vi "Main.vi"() -> ()   [LabVIEW 2017, in "Eulogy.lvlib" / "Bookmark Manager.lvlib"]
uses:
  Bookmark Manager.lvlib
  Private/State.ctl
panel:
  in  "Help":bool
  in  "Close":bool
  in  "Tomestones":string(tree)
  in  "Scope":u16(ring)
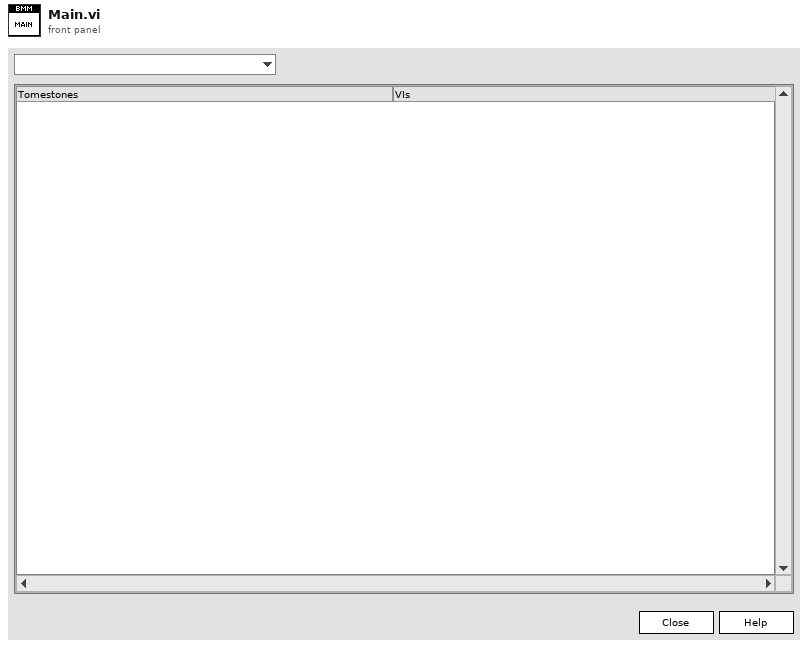
[diagram p1: front panel]
types:
  T1 = typedef "Eulogy.lvlib/Bookmark Manager.lvlib/State.ctl" = cluster{"Projects":refnum<vi>, "Tree":refnum<vi>, "Front Panel":refnum<vi>}
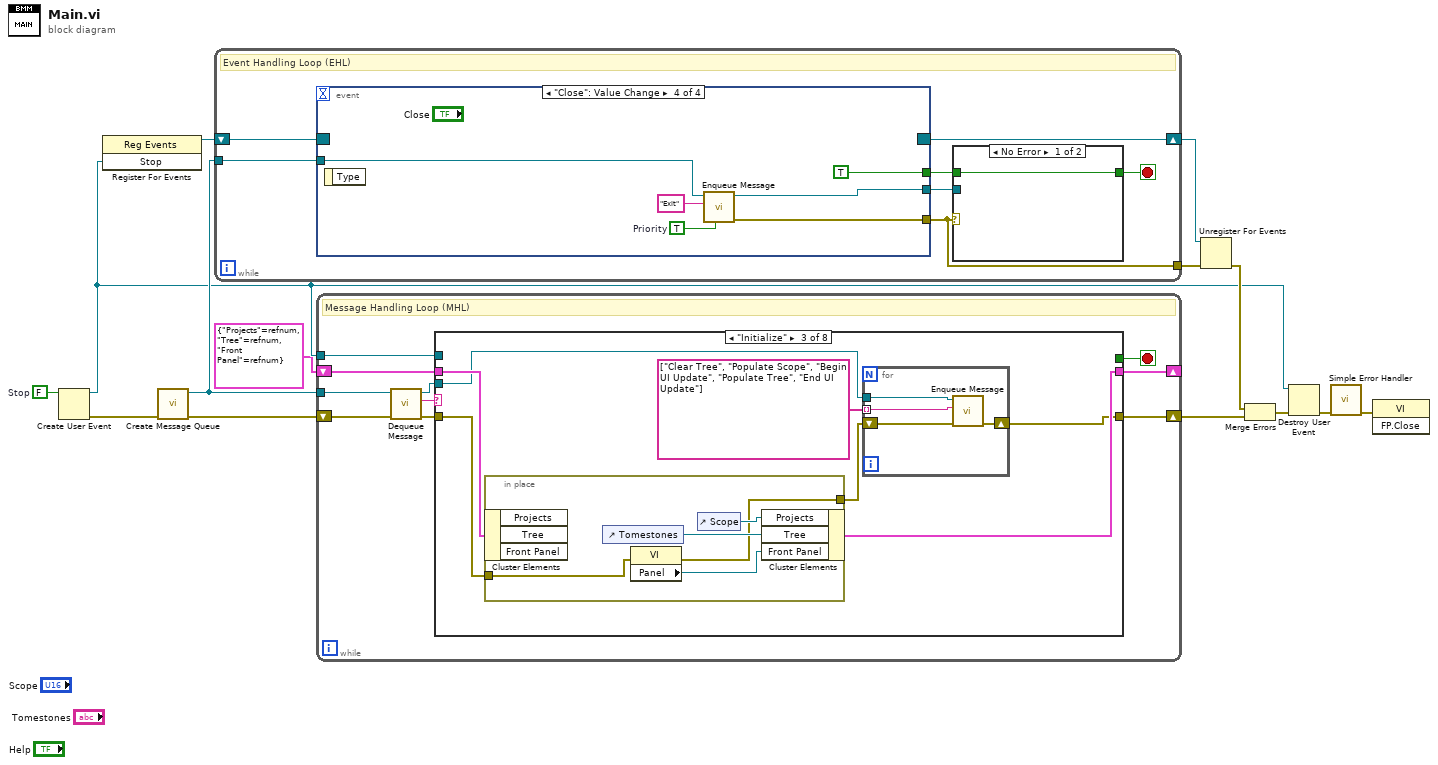
[diagram p0: block diagram]
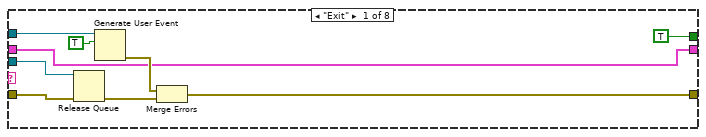
[diagram p2: hidden frame]
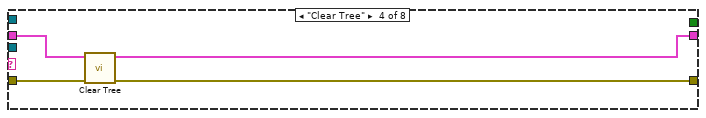
[diagram p4: hidden frame]
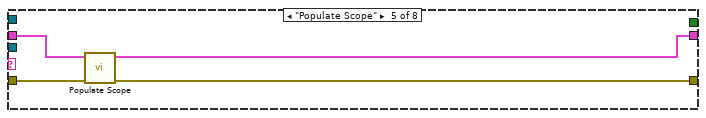
[diagram p5: hidden frame]
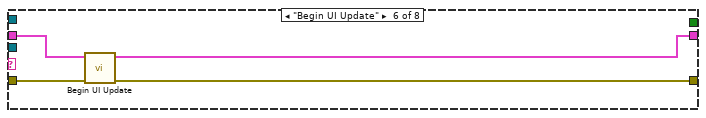
[diagram p6: hidden frame]
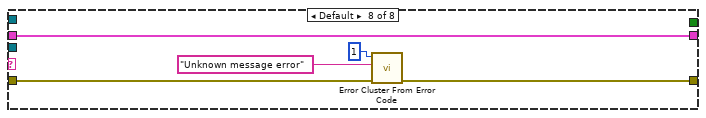
[diagram p8: hidden frame]
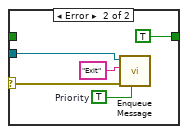
[diagram p9: hidden frame]
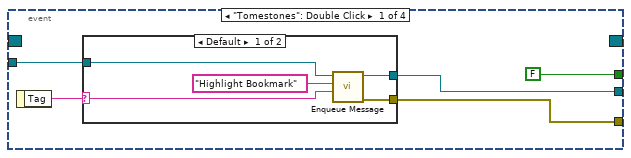
[diagram p10: hidden frame]
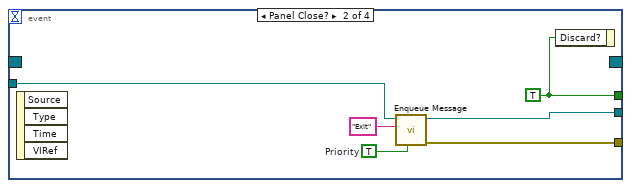
[diagram p12: hidden frame]
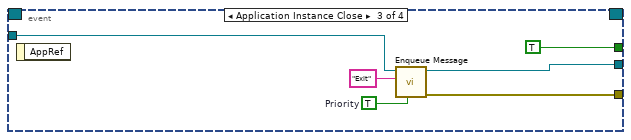
[diagram p13: hidden frame]
diagram:
  w11 = FALSE  # Stop
  n1 = Create User Event(user event datatype=w11) -> (user event=w4:refnum<user-event>, error out=w10:errorcluster)  [unwired: 1 in]
  n2 = register-events(w4) -> (reference out=w14:refnum<event-registration>)  [unwired: 2 in, 1 out]
  n3 = call "Create Message Queue.vi"("Error In"=w10) -> ("Error Out"=w8:errorcluster, "Message Queue"=w9:refnum<queue>)  [unwired: 9 in]
  n4 = while {
    shift-right: [w20] -> w13
    shift-left: w14 -> [w21]
    tunnel: [w17] -> w12
    tunnel: w9 -> [w15]
    stop <- w18 stop-if-true
    # "Event Handling Loop (EHL)"
    n5 = event shown="[3] \"Close\": Value Change" {
      selector: w21 -> [_ _ _ _]
      dyn-events: [_ _ _ _] -> w20
      timeout: _ -> [_ _ _ _]
      tunnel: [w32 w42 w49 w55] -> w17
      tunnel: [FALSE w44 TRUE TRUE] -> w19
      tunnel: [w30 w43 w50 w56] -> w16
      tunnel: w15 -> [w28 w39 w46 w52]
      event "Tomestones": Double Click {
        n6 = event-data() -> ("Tag"=w29:string)  [unwired: 1 in]
        n7 = case shown="Default" w29 {
          selector: w29 -> [w34 _]
          tunnel: [w36 _] -> w32
          tunnel: [w37 w38] -> w30
          tunnel: w28 -> [w33 w38]
          frame Default {
            n8 = call "Enqueue Message.vi"("Data"=w34, "Command"="Highlight Bookmark", "Message Queue In"=w33) -> ("Error Out"=w36:errorcluster, "Message Queue Out"=w37:refnum<queue>)  [unwired: 7 in]
          }
          frame "" {
          }
        }
      }
      event Panel Close? {
        w40 = TRUE  # Priority
        w44 = TRUE
        n9 = event-data() -> ()  [unwired: 1 in, 4 out]
        n10 = call "Enqueue Message.vi"("Priority"=w40, "Command"="Exit", "Message Queue In"=w39) -> ("Error Out"=w42:errorcluster, "Message Queue Out"=w43:refnum<queue>)  [unwired: 7 in]
        n11 = event-data("Discard?"=w44) -> ()  [unwired: 1 in, 1 out]
      }
      event Application Instance Close {
        w47 = TRUE  # Priority
        n12 = event-data() -> ()  [unwired: 1 in, 1 out]
        n13 = call "Enqueue Message.vi"("Priority"=w47, "Command"="Exit", "Message Queue In"=w46) -> ("Error Out"=w49:errorcluster, "Message Queue Out"=w50:refnum<queue>)  [unwired: 7 in]
      }
      event "Close": Value Change {
        w53 = TRUE  # Priority
        n14 = event-data() -> ()  [unwired: 1 in, 1 out]
        n15 = call "Enqueue Message.vi"("Priority"=w53, "Command"="Exit", "Message Queue In"=w52) -> ("Error Out"=w55:errorcluster, "Message Queue Out"=w56:refnum<queue>)  [unwired: 7 in]
      }
    }
    n16 = case shown="No Error" w17 {
      selector: w17 -> [_ w27]
      tunnel: w19 -> [w22 _]
      tunnel: [w22 TRUE] -> w18
      tunnel: w16 -> [_ w25]
      frame No Error {
      }
      frame Error {
        w23 = TRUE  # Priority
        n17 = call "Enqueue Message.vi"("Priority"=w23, "Error In"=w27, "Command"="Exit", "Message Queue In"=w25) -> ()  [unwired: 6 in, 2 out]
      }
    }
  }
  n18 = while {
    tunnel: w9 -> [w66]
    shift-right: [w64] -> w6
    shift-left: w8 -> [w63]
    tunnel: w4 -> [w60]
    shift-right: [w57] -> _
    shift-left: T1 {"Projects"=refnum, "Tree"=refnum, "Front Panel"=refnum} ("State") -> [w58]
    stop <- w61 stop-if-true
    # "Message Handling Loop (MHL)"
    n19 = call "Dequeue Message.vi"("Error In"=w63, "Message Queue In"=w66) -> ("Error Out"=w62:errorcluster, "Command"=w65:string, "Message Queue Out"=w59:refnum<queue>)  [unwired: 6 in, 1 out]
    n20 = case shown="\"Initialize\"" w65 {
      tunnel: [w73 w77 w81 w94 w98 w103 w107 w108] -> w64
      tunnel: w62 -> [w75 w77 w80 w95 w99 w102 w107 w110]
      tunnel: [TRUE _ _ _ _ _ _ _] -> w61
      tunnel: w60 -> [w72 _ _ _ _ _ _ _]
      tunnel: w59 -> [w68 _ w82 _ _ _ _ _]
      tunnel: w58 -> [w67 w76 w84 w97 w101 w105 w106 w109]
      tunnel: [w67 w76 w83 w96 w100 w104 w106 w109] -> w57
      frame "Exit" {
        n21 = Release Queue(queue=w68, error in (no error)=w75) -> (error out=w69:errorcluster)  [unwired: 1 in, 2 out]
        n22 = Generate User Event(user event=w72, event data cluster=TRUE ("event data")) -> (error out=w70:errorcluster)  [unwired: 2 in, 1 out]
        n23 = Merge Errors(w70, w69) -> (w73:errorcluster)
      }
      frame "Highlight Bookmark" {
      }
      frame "Initialize" {
        n24 = in-place {
          in-place-border: w80 -> [w90]
          in-place-border: [w89] -> w79
          n25 = in-place-cluster #1(w84) -> ()  [unwired: 3 out]
          n26 = control-ref of="Tomestones"() -> (w92:refnum<vi>)
          n27 = property class="VI"(error in=w90) -> (error out=w89:errorcluster, "Panel"=w91:refnum<vi>)  [unwired: 1 in, 1 out]
          n28 = control-ref of="Scope"() -> (w93:refnum<vi>)
          n29 = in-place-cluster #1("Projects"=w93, "Tree"=w92, "Front Panel"=w91) -> (w83:T1)
        }
        n30 = for {
          tunnel: w82 -> [w88]
          shift-right: [w87] -> w81
          shift-left: w79 -> [w86]
          tunnel: string[] ["Clear Tree", "Populate Scope", "Begin UI Update", "Populate Tree", "End UI Update"] -> [w85] mode=indexing
          n31 = call "Enqueue Message.vi"("Error In"=w86, "Command"=w85, "Message Queue In"=w88) -> ("Error Out"=w87:errorcluster)  [unwired: 7 in, 1 out]
        }
      }
      frame "Clear Tree" {
        n32 = call "Clear Tree.vi"("Error In"=w95, "State In"=w97) -> ("Error Out"=w94:errorcluster, "State Out"=w96:T1)  [unwired: 8 in]
      }
      frame "Populate Scope" {
        n33 = call "Populate Scope.vi"("Error In"=w99, "State In"=w101) -> ("Error Out"=w98:errorcluster, "State Out"=w100:T1)  [unwired: 8 in]
      }
      frame "Begin UI Update" {
        n34 = call "Begin UI Update.vi"("Error In"=w102, "State In"=w105) -> ("Error Out"=w103:errorcluster, "State Out"=w104:T1)  [unwired: 8 in]
      }
      frame "Populate Tree" {
      }
      frame Default {
        n35 = call <vilib>:"Error Cluster From Error Code.vi"("error in (no error)"=w110, "error message (\"\")"="Unknown message error" ("error message (\"\")"), "error code (0)"=1) -> ("error out"=w108:errorcluster)  [unwired: 6 in]
      }
    }
  }
  n36 = Unregister For Events(event registration refnum=w13, error in=w12) -> (error out=w7:errorcluster)
  n37 = Merge Errors(w7, w6) -> (w5:errorcluster)
  n38 = Destroy User Event(user event=w4, error in=w5) -> (error out=w3:errorcluster)
  n39 = call <vilib>:"Simple Error Handler.vi"("error in (no error)"=w3) -> ("error out"=w2:errorcluster)  [unwired: 4 in, 4 out]
  n40 = invoke class="VI" method="FP.Close"(error in=w2) -> ()  [unwired: 2 in, 3 out]
